vi "dn24f08.vi"() -> ()   [LabVIEW 2015]
uses:
  <vilib>/Instr/_visa.llb/VISA Configure Serial Port (Instr).vi
panel:
  out "engineExit":bool
  out "guiExit":bool
  in  "exit":bool
  out "analogValue":dbl
  in  "getAnalog":bool
  in  "analogInput":u8
  out "inputState":bool
  in  "outputState":bool
  in  "getPin":bool
  in  "digitalInput":u8
  in  "setPin":bool
  in  "digitalOutput":u8
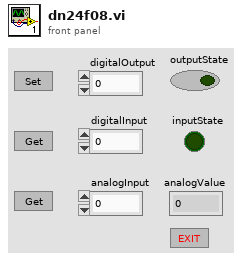
[diagram p1: front panel]
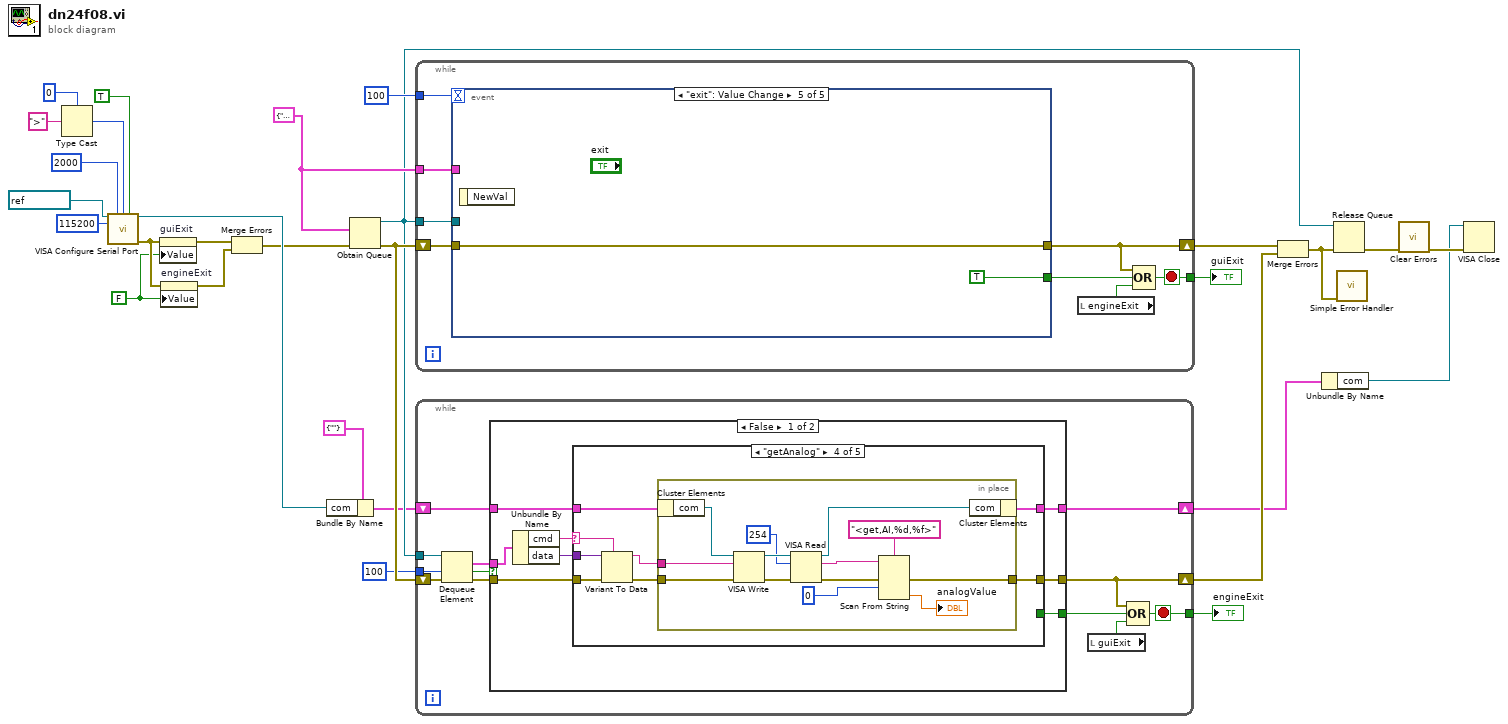
[diagram p0: block diagram]
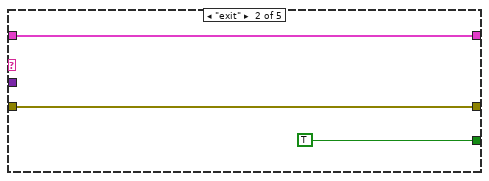
[diagram p3: hidden frame]
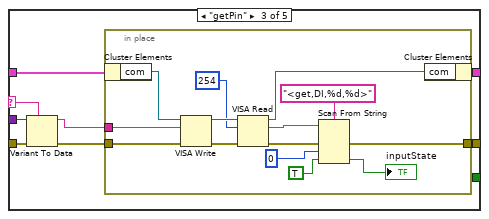
[diagram p4: hidden frame]
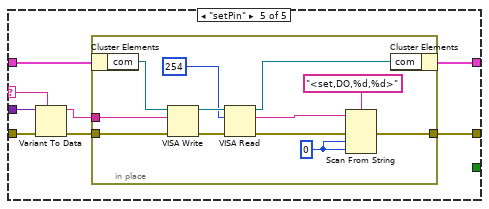
[diagram p5: hidden frame]
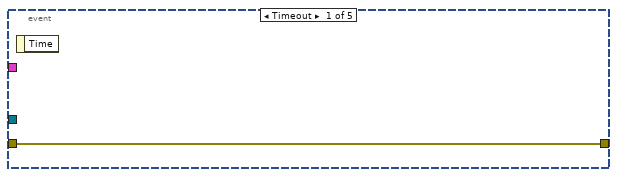
[diagram p7: hidden frame]
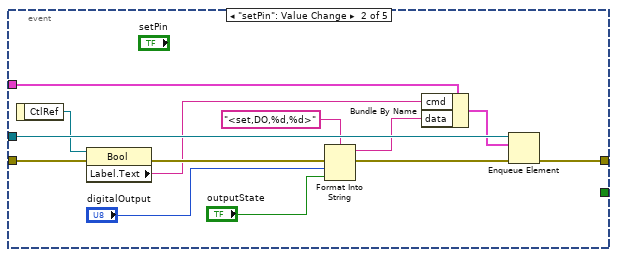
[diagram p8: hidden frame]
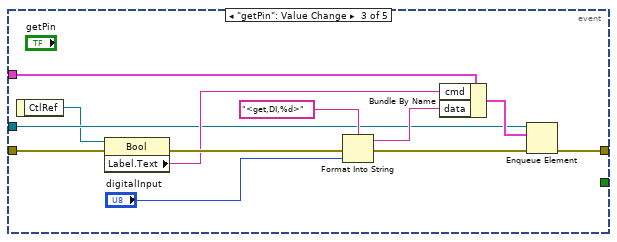
[diagram p9: hidden frame]
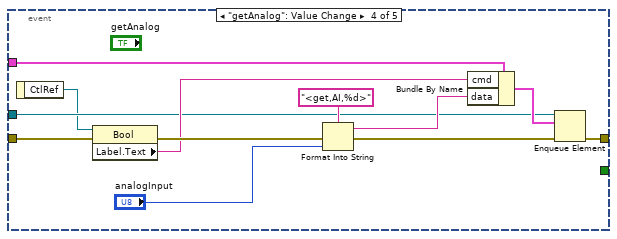
[diagram p10: hidden frame]
diagram:
  w1 = FALSE ("guiExit")
  w26 = cluster{"cmd":string, "data":variant} {"cmd"="", "data"=variant}
  n1 = Type Cast(type=u8 0, x=">") -> (*(type *) &x=w19:u8)
  n2 = call-poly "VISA Configure Serial Port"("VISA resource name"=refnum<visa-resource-name> "COM7", "timeout (10sec)"=u32 2000, "termination char\n(0xA = '\\n' = LF)"=w19, "Enable Termination\nChar (T)"=TRUE ("Enable Termination\nChar (T)"), "baud rate (9600)"=u32 115200) -> ("VISA resource name out"=w20:refnum<visa-resource-name>, "error out"=w5:errorcluster)  [unwired: 9 in]
  n3 = property on="guiExit" class="Bool (strict)"(error in=w5, "Value"=w1) -> (error out=w4:errorcluster)  [unwired: 1 in, 1 out]
  n4 = property on="engineExit" class="Bool (strict)"(error in=w5, "Value"=w1) -> (error out=w3:errorcluster)  [unwired: 1 in, 1 out]
  n5 = Merge Errors(w4, w3) -> (w2:errorcluster)
  n6 = Bundle By Name(cluster=cluster{"com":refnum<visa-resource-name>} {"com"=""}, "com"=w20) -> (w21:cluster{"com":refnum<visa-resource-name>})
  n7 = Obtain Queue(element data type=w26, error in (no error)=w2) -> (queue out=w23:refnum<queue>, error out=w29:errorcluster)  [unwired: 3 in, 1 out]
  n8 = while {
    tunnel: w23 -> [w35]
    shift-right: [w32] -> w25
    shift-left: w29 -> [w37]
    tunnel: 100 -> [w36]
    tunnel: w26 -> [w34]
    tunnel: [w33] -> w7
    stop <- w33 stop-if-true
    n9 = event shown="[4] \"exit\": Value Change" {
      selector: _ -> [_ _ _ _ _]
      dyn-events: _ -> [_ _ _ _ _]
      timeout: w36 -> [_ _ _ _ _]
      tunnel: w37 -> [w38 w47 w57 w67 w77]
      tunnel: [w38 w51 w52 w65 w77] -> w32
      tunnel: w35 -> [_ w50 w56 w69 _]
      tunnel: [_ _ _ _ TRUE] -> w31
      tunnel: w34 -> [_ w49 w54 w68 _]
      event Timeout {
        n10 = event-data() -> ()  [unwired: 1 in, 1 out]
      }
      event "setPin": Value Change {
        n11 = event-data() -> ("CtlRef"=w46:refnum<vi>)  [unwired: 1 in]
        n12 = property class="Bool"(reference=w46, error in=w47) -> (error out=w45:errorcluster, "Label.Text"=w44:string)  [unwired: 1 out]
        n13 = Format Into String(format string="<set,DO,%d,%d>", error in=w45, "digitalOutput", "outputState") -> (resulting string=w39:string, error out=w43:errorcluster)  [unwired: 1 in]
        n14 = Bundle By Name(cluster=w49, "cmd"=w44, "data"=w39) -> (w48:cluster{"cmd":string, "data":variant})
        n15 = Enqueue Element(queue=w50, element=w48, error in (no error)=w43) -> (error out=w51:errorcluster)  [unwired: 1 in, 2 out]
      }
      event "getPin": Value Change {
        n16 = event-data() -> ("CtlRef"=w55:refnum<vi>)  [unwired: 1 in]
        n17 = property class="Bool"(reference=w55, error in=w57) -> (error out=w62:errorcluster, "Label.Text"=w61:string)  [unwired: 1 out]
        n18 = Format Into String(format string="<get,DI,%d>", error in=w62, "digitalInput") -> (resulting string=w58:string, error out=w60:errorcluster)  [unwired: 1 in]
        n19 = Bundle By Name(cluster=w54, "cmd"=w61, "data"=w58) -> (w63:cluster{"cmd":string, "data":variant})
        n20 = Enqueue Element(queue=w56, element=w63, error in (no error)=w60) -> (error out=w52:errorcluster)  [unwired: 1 in, 2 out]
      }
      event "getAnalog": Value Change {
        n21 = event-data() -> ("CtlRef"=w66:refnum<vi>)  [unwired: 1 in]
        n22 = property class="Bool"(reference=w66, error in=w67) -> (error out=w74:errorcluster, "Label.Text"=w73:string)  [unwired: 1 out]
        n23 = Format Into String(format string="<get,AI,%d>", error in=w74, "analogInput") -> (resulting string=w70:string, error out=w72:errorcluster)  [unwired: 1 in]
        n24 = Bundle By Name(cluster=w68, "cmd"=w73, "data"=w70) -> (w75:cluster{"cmd":string, "data":variant})
        n25 = Enqueue Element(queue=w69, element=w75, error in (no error)=w72) -> (error out=w65:errorcluster)  [unwired: 1 in, 2 out]
      }
      event "exit": Value Change {
        n26 = event-data() -> ()  [unwired: 1 in, 1 out]
      }
    }
    n27 = local read "engineExit"() -> (w30:bool)
    n28 = Compound Arithmetic op=OR(w32, w31, w30) -> (w33:bool)
  }
  "guiExit" <- w7
  n29 = while {
    tunnel: w23 -> [w88]
    shift-right: [w80] -> w24
    shift-left: w29 -> [w87]
    tunnel: 100 ("timeout in ms (-1)") -> [w84]
    shift-right: [w82] -> w10
    shift-left: w21 -> [w83]
    tunnel: [w81] -> w8
    stop <- w81 stop-if-true
    n30 = Dequeue Element(queue=w88, timeout in ms (-1)=w84, error in (no error)=w87) -> (element=w85:cluster{"cmd":string, "data":variant}, timed out?=w89:bool, error out=w86:errorcluster)  [unwired: 1 out]
    n31 = case shown="False" w89 {
      tunnel: [w92 w167] -> w80
      tunnel: w86 -> [w94 w167]
      tunnel: w85 -> [w97 _]
      tunnel: w83 -> [w93 w166]
      tunnel: [w91 w166] -> w82
      tunnel: [w90 _] -> w79
      frame False {
        n32 = Unbundle By Name(w97) -> ("cmd"=w96:string, "data"=w95:variant)
        n33 = case shown="\"getAnalog\"" w96 {
          selector: w96 -> [_ _ w108 w128 w149]
          tunnel: w95 -> [_ _ w109 w129 w151]
          tunnel: w94 -> [w98 w101 w110 w130 w150]
          tunnel: w93 -> [w99 w102 w107 w127 w148]
          tunnel: [w98 w101 w104 w125 w146] -> w92
          tunnel: [w99 w102 w103 w126 w147] -> w91
          tunnel: [_ TRUE _ _ _] -> w90
          frame "False", Default {
          }
          frame "exit" {
          }
          frame "getPin" {
            n34 = Variant To Data(error in=w110, type=w108, Variant=w109) -> (data=w105:string, error out=w106:errorcluster)
            n35 = in-place {
              in-place-border: w106 -> [w124]
              in-place-border: w105 -> [w123]
              in-place-border: [w121] -> w104
              n36 = in-place-cluster #1(w107) -> ("com"=w122:refnum<visa-resource-name>)
              n37 = VISA Write(VISA resource name=w122, write buffer=w123, error in (no error)=w124) -> (VISA resource name out=w116:refnum<visa-resource-name>, error out=w118:errorcluster)  [unwired: 1 out]
              n38 = VISA Read(VISA resource name=w116, byte count=u32 254, error in (no error)=w118) -> (VISA resource name out=w115:refnum<visa-resource-name>, read buffer=w114:string, error out=w117:errorcluster)  [unwired: 1 out]
              n39 = Scan From String(format string="<get,DI,%d,%d>", input string=w114, error in=w117, default 1=u8 0 ("default value 2"), default 2=TRUE) -> (error out=w121:errorcluster, output 2=→"inputState":bool)  [unwired: 2 in, 2 out]
              n40 = in-place-cluster #1("com"=w115) -> (w103:cluster{"com":refnum<visa-resource-name>})
            }
          }
          frame "getAnalog" {
            n41 = Variant To Data(error in=w130, type=w128, Variant=w129) -> (data=w131:string, error out=w132:errorcluster)
            n42 = in-place {
              in-place-border: w132 -> [w145]
              in-place-border: w131 -> [w144]
              in-place-border: [w142] -> w125
              n43 = in-place-cluster #2(w127) -> ("com"=w143:refnum<visa-resource-name>)
              n44 = VISA Write(VISA resource name=w143, write buffer=w144, error in (no error)=w145) -> (VISA resource name out=w137:refnum<visa-resource-name>, error out=w139:errorcluster)  [unwired: 1 out]
              n45 = VISA Read(VISA resource name=w137, byte count=u32 254, error in (no error)=w139) -> (VISA resource name out=w136:refnum<visa-resource-name>, read buffer=w135:string, error out=w138:errorcluster)  [unwired: 1 out]
              n46 = Scan From String(format string="<get,AI,%d,%f>", input string=w135, error in=w138, default 1=u8 0 ("default value 2")) -> (error out=w142:errorcluster, output 2=→"analogValue":dbl)  [unwired: 3 in, 2 out]
              n47 = in-place-cluster #2("com"=w136) -> (w126:cluster{"com":refnum<visa-resource-name>})
            }
          }
          frame "setPin" {
            n48 = Variant To Data(error in=w150, type=w149, Variant=w151) -> (data=w152:string, error out=w153:errorcluster)
            n49 = in-place {
              in-place-border: w153 -> [w165]
              in-place-border: w152 -> [w164]
              in-place-border: [w162] -> w146
              w155 = u8 0 ("default value 2")
              n50 = in-place-cluster #3(w148) -> ("com"=w163:refnum<visa-resource-name>)
              n51 = VISA Write(VISA resource name=w163, write buffer=w164, error in (no error)=w165) -> (VISA resource name out=w158:refnum<visa-resource-name>, error out=w160:errorcluster)  [unwired: 1 out]
              n52 = VISA Read(VISA resource name=w158, byte count=u32 254, error in (no error)=w160) -> (VISA resource name out=w157:refnum<visa-resource-name>, read buffer=w156:string, error out=w159:errorcluster)  [unwired: 1 out]
              n53 = Scan From String(format string="<set,DO,%d,%d>", input string=w156, error in=w159, default 1=w155, default 2=w155) -> (error out=w162:errorcluster)  [unwired: 3 in, 2 out]
              n54 = in-place-cluster #3("com"=w157) -> (w147:cluster{"com":refnum<visa-resource-name>})
            }
          }
        }
      }
      frame True {
      }
    }
    n55 = local read "guiExit"() -> (w78:bool)
    n56 = Compound Arithmetic op=OR(w80, w79, w78) -> (w81:bool)
  }
  "engineExit" <- w8
  n57 = Merge Errors(w25, w24) -> (w6:errorcluster)
  n58 = Unbundle By Name(w10) -> ("com"=w9:refnum<visa-resource-name>)
  n59 = Release Queue(queue=w23, error in (no error)=w6) -> (error out=w12:errorcluster)  [unwired: 1 in, 2 out]
  n60 = call <vilib>:"Simple Error Handler.vi"("error in (no error)"=w6) -> ()  [unwired: 4 in, 5 out]
  n61 = call <vilib>:"Clear Errors.vi"("error in (no error)"=w12) -> ("error out"=w11:errorcluster)  [unwired: 5 in, 1 out]
  n62 = VISA Close(VISA resource name=w9, error in (no error)=w11) -> ()  [unwired: 1 out]
